vi "Joystick tuner.vi"(0 "Joystick Z":dbl, 3 "Loop ID":i32, 4 "Max":dbl=1.5, 8 "Min":dbl=0.25) -> (7 "Output":dbl)   [LabVIEW 2013]
panel:
  # "a reentrant joystick tuning utility"
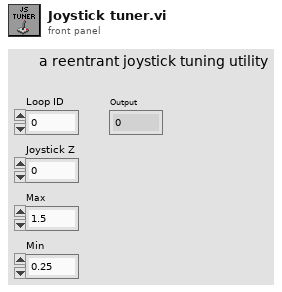
[diagram p1: front panel]
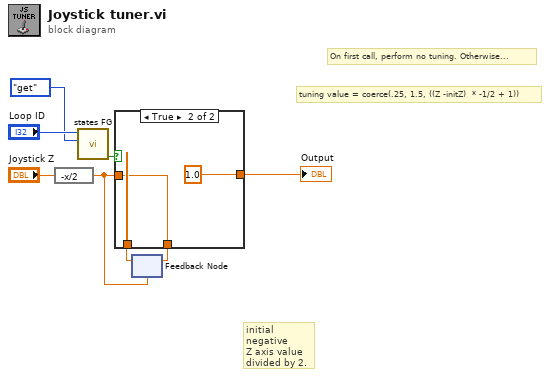
[diagram p0: block diagram]
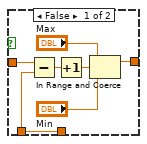
[diagram p2: hidden frame]
diagram:
  # "tuning value = coerce(.25, 1.5, ((Z -initZ)  * -1/2 + 1))"
  # "initial negative\nZ axis value\ndivided by 2."
  # "On first call, perform no tuning. Otherwise..."
  n1 = expression code="-x/2"("Joystick Z") -> (w4:dbl)
  n2 = call "states FG.vi"("menu (get)"=enum16{"set", "get"}."get", "Loop ID"="Loop ID") -> ("first call?"=w6:bool)  [unwired: 6 in, 3 out]
  n3 = feedback #1(w4) -> (w8:dbl)
  n4 = case shown="True" w6 {
    tunnel: w4 -> [w15 w17]
    tunnel: [w12 w17] -> w7
    tunnel: w8 -> [w12 _]
    tunnel: [w14 1.0 ("upper limit")] -> w2
    frame False {
      n5 = Subtract(x=w15, y=w12) -> (x-y=w13:dbl)
      n6 = Increment(x=w13) -> (x+1=w11:dbl)
      n7 = In Range and Coerce(upper limit="Max", x=w11, lower limit="Min") -> (coerced(x)=w14:dbl)  [unwired: 1 out]
    }
    frame True {
    }
  }
  "Output" <- w2
  n8 = feedback-in #1(w7) -> ()
